vi "String_Count.vi"() -> ()   [LabVIEW 2019]
panel:
  out "length":i32
  in  "String":string
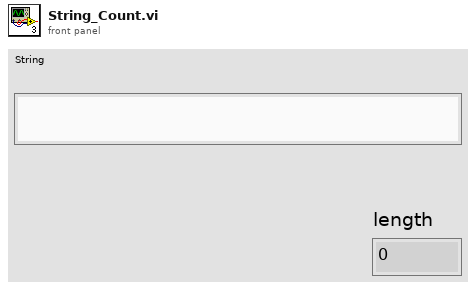
[diagram p1: front panel]
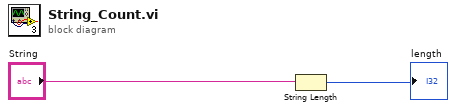
[diagram p0: block diagram]
diagram:
  n1 = String Length(string="String") -> (length=→"length":i32)
